vi "kousei - Response Parser.vi"(8 "error in (no error)":errorcluster, 10 "body":string, 11 "headers":string) -> (0 "error out":errorcluster, 3 "Response":T1)   [LabVIEW 2015, in "LV-Proof-Reading.lvlib"]
uses:
  LV-Proof-Reading.lvlib
  kousei - Response Data JSON.ctl
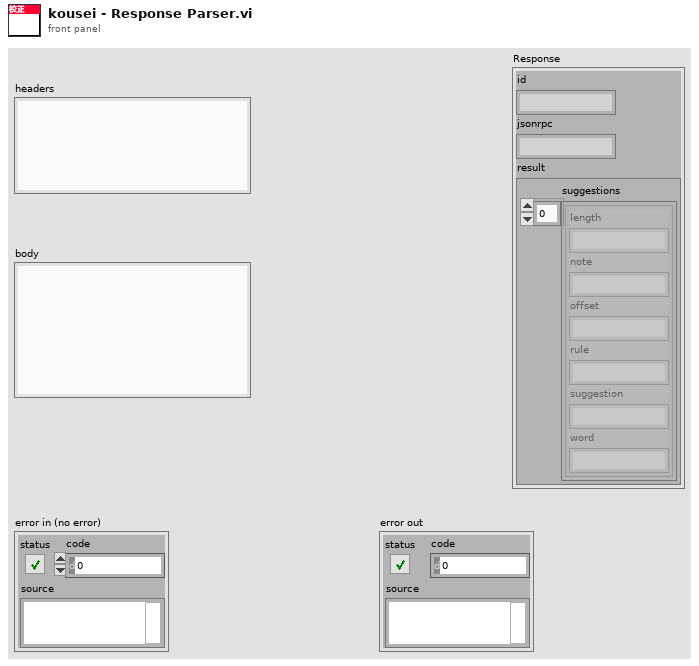
[diagram p1: front panel]
types:
  T1 = typedef "LV-Proof-Reading.lvlib/kousei - Response Data JSON.ctl" = cluster{"id":string, "jsonrpc":string, "result":cluster{"suggestions":cluster{"length":string, "note":string, "offset":string, "rule":string, "suggestion":string, "word":string}[]}}
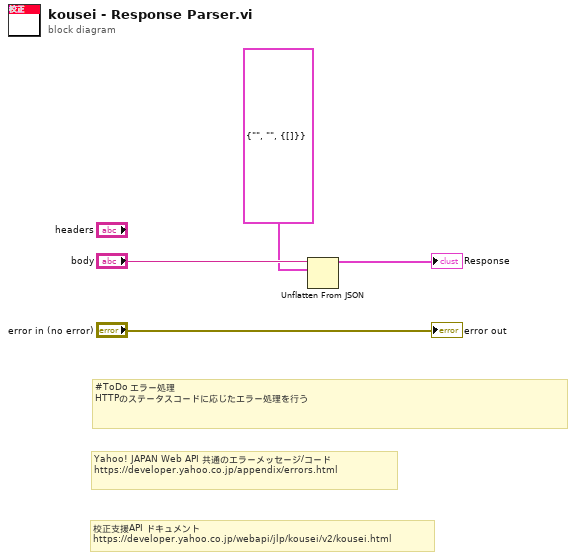
[diagram p0: block diagram]
diagram:
  # "Yahoo! JAPAN Web API 共通のエラーメッセージ/コード\nhttps://developer.yahoo.co.jp/appendix/errors.html"
  # "校正支援API ドキュメント\nhttps://developer.yahoo.co.jp/webapi/jlp/kousei/v2/kousei.html"
  # "#ToDo エラー処理 \nHTTPのステータスコードに応じたエラー処理を行う"
  n1 = Unflatten From JSON(JSON string="body", type and defaults=T1 {"id"="", "jsonrpc"="", "result"={"suggestions"=[]}} ("Root")) -> (value=→"Response":T1)  [unwired: 5 in, 1 out]
  "error out" <- "error in (no error)"
